vi "buildTestLog.vi"(8 "error in (no error)":errorcluster, 9 "Serial Number":string, 10 "TestLogTypes":T1, 11 "ITestLogFactory in":refnum<class "ITestLogFactory.lvclass">) -> (0 "error out":errorcluster, 2 "ITestLog.lvclass":refnum<class "ITestLog.lvclass">, 3 "ITestLogFactory out":refnum<class "ITestLogFactory.lvclass">)   [LabVIEW 2015, in "ITestLogFactory.lvclass"]
uses:
  ITestLogFactory.lvclass
  Typedefs/TestLogTypes.ctl
  TestLog/ITestLog/ITestLog.lvclass
  Typedefs/ILCBTTypedefs.lvlib
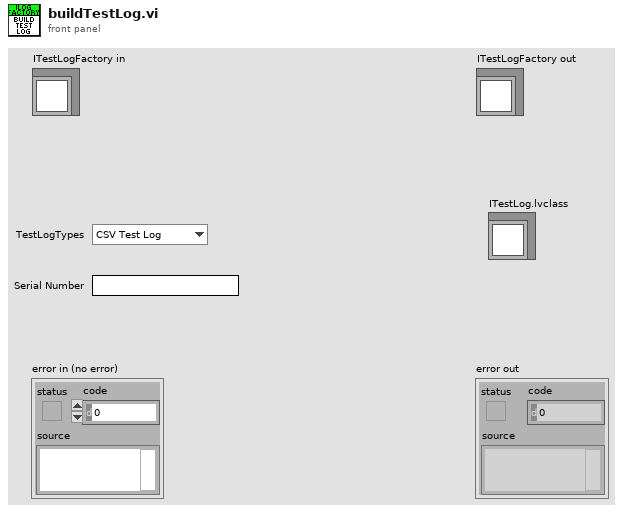
[diagram p1: front panel]
types:
  T1 = typedef "ILCBTTypedefs.lvlib/TestLogTypes.ctl" = enum16{"CSV Test Log"}
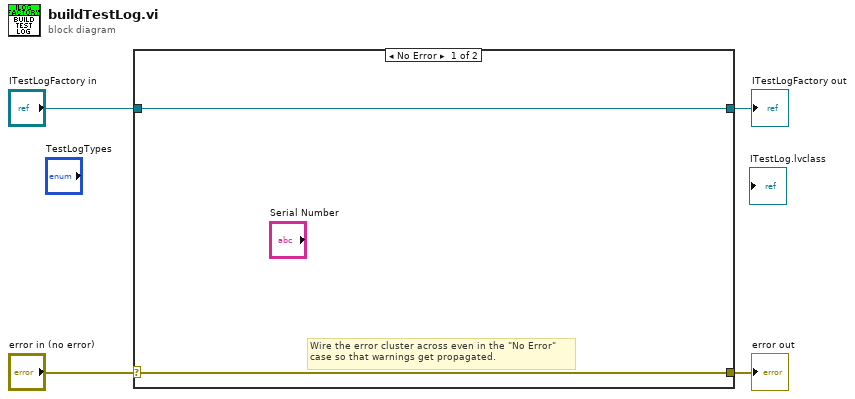
[diagram p0: block diagram]
diagram:
  n1 = case shown="No Error" "error in (no error)" {
    selector: "error in (no error)" -> [w5 w8]
    tunnel: [w5 w8] -> w3
    tunnel: [w6 w7] -> w1
    tunnel: "ITestLogFactory in" -> [w6 w7]
    frame No Error {
      # "Wire the error cluster across even in the \"No Error\"\ncase so that warnings get propagated."
    }
    frame Error {
    }
  }
  "error out" <- w3
  "ITestLogFactory out" <- w1
